vi "PID Table (Ultimate Gain and Frequency - Ziegler Nichols).vi"(5 "Control Design":u16(ring) items=["Fast", "Normal", "Slow"], 7 "Type of Controller":u16(ring)=1 items=["P", "PI", "PID"], 10 "Ultimate Period (Tu)":dbl, 11 "Ultimate Gain (Ku)":dbl) -> (1 "Derivative Time (Td)":dbl, 2 "Integral Time (Ti)":dbl, 3 "Proportional Gain (Kp)":dbl)   [LabVIEW 2017]
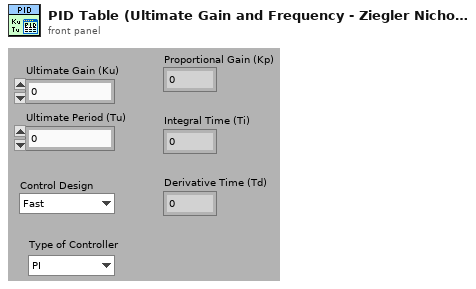
[diagram p1: front panel]
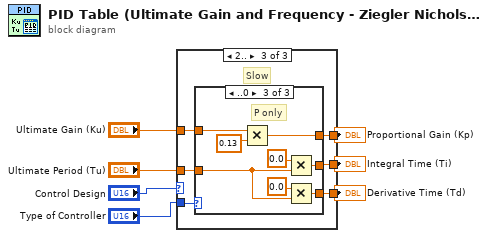
[diagram p0: block diagram]
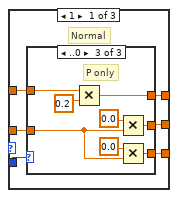
[diagram p2: hidden frame]
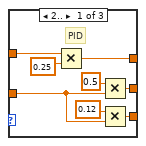
[diagram p3: hidden frame]
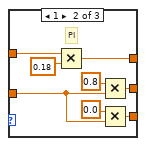
[diagram p4: hidden frame]
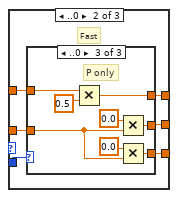
[diagram p5: hidden frame]
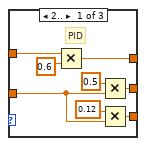
[diagram p6: hidden frame]
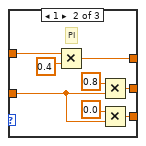
[diagram p7: hidden frame]
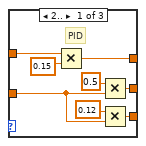
[diagram p8: hidden frame]
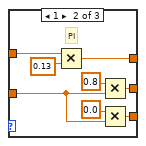
[diagram p9: hidden frame]
diagram:
  n1 = case shown="2.." "Control Design" {
    tunnel: [w13 w43 w73] -> w6
    tunnel: [w12 w42 w72] -> w7
    tunnel: [w11 w41 w71] -> w5
    tunnel: "Ultimate Period (Tu)" -> [w10 w40 w70]
    tunnel: "Ultimate Gain (Ku)" -> [w9 w39 w69]
    tunnel: "Type of Controller" -> [w8 w38 w68]
    frame 1 {
      # "Normal"
      n2 = case shown="..0" w8 {
        tunnel: [w14 w22 w30] -> w11
        tunnel: [w19 w27 w35] -> w13
        tunnel: w10 -> [w18 w26 w34]
        tunnel: [w15 w23 w31] -> w12
        tunnel: w9 -> [w16 w24 w32]
        frame 2.. {
          # "PID"
          n3 = Multiply(x=w16, y=0.25) -> (x*y=w14:dbl)
          n4 = Multiply(x=0.5, y=w18) -> (x*y=w15:dbl)
          n5 = Multiply(x=0.12, y=w18) -> (x*y=w19:dbl)
        }
        frame 1 {
          # "PI"
          n6 = Multiply(x=w24, y=0.18) -> (x*y=w22:dbl)
          n7 = Multiply(x=0.8, y=w26) -> (x*y=w23:dbl)
          n8 = Multiply(x=0.0, y=w26) -> (x*y=w27:dbl)
        }
        frame ..0 {
          # "P only"
          n9 = Multiply(x=w32, y=0.2) -> (x*y=w30:dbl)
          n10 = Multiply(x=0.0, y=w34) -> (x*y=w31:dbl)
          n11 = Multiply(x=0.0, y=w34) -> (x*y=w35:dbl)
        }
      }
    }
    frame ..0 {
      # "Fast"
      n12 = case shown="..0" w38 {
        tunnel: [w44 w52 w60] -> w41
        tunnel: [w49 w57 w65] -> w43
        tunnel: w40 -> [w48 w56 w64]
        tunnel: [w45 w53 w61] -> w42
        tunnel: w39 -> [w46 w54 w62]
        frame 2.. {
          # "PID"
          n13 = Multiply(x=w46, y=0.6) -> (x*y=w44:dbl)
          n14 = Multiply(x=0.5, y=w48) -> (x*y=w45:dbl)
          n15 = Multiply(x=0.12, y=w48) -> (x*y=w49:dbl)
        }
        frame 1 {
          # "PI"
          n16 = Multiply(x=w54, y=0.4) -> (x*y=w52:dbl)
          n17 = Multiply(x=0.8, y=w56) -> (x*y=w53:dbl)
          n18 = Multiply(x=0.0, y=w56) -> (x*y=w57:dbl)
        }
        frame ..0 {
          # "P only"
          n19 = Multiply(x=w62, y=0.5) -> (x*y=w60:dbl)
          n20 = Multiply(x=0.0, y=w64) -> (x*y=w61:dbl)
          n21 = Multiply(x=0.0, y=w64) -> (x*y=w65:dbl)
        }
      }
    }
    frame 2.. {
      # "Slow"
      n22 = case shown="..0" w68 {
        tunnel: [w74 w82 w90] -> w71
        tunnel: [w79 w87 w95] -> w73
        tunnel: w70 -> [w78 w86 w94]
        tunnel: [w75 w83 w91] -> w72
        tunnel: w69 -> [w76 w84 w92]
        frame 2.. {
          # "PID"
          n23 = Multiply(x=w76, y=0.15) -> (x*y=w74:dbl)
          n24 = Multiply(x=0.5, y=w78) -> (x*y=w75:dbl)
          n25 = Multiply(x=0.12, y=w78) -> (x*y=w79:dbl)
        }
        frame 1 {
          # "PI"
          n26 = Multiply(x=w84, y=0.13) -> (x*y=w82:dbl)
          n27 = Multiply(x=0.8, y=w86) -> (x*y=w83:dbl)
          n28 = Multiply(x=0.0, y=w86) -> (x*y=w87:dbl)
        }
        frame ..0 {
          # "P only"
          n29 = Multiply(x=w92, y=0.13) -> (x*y=w90:dbl)
          n30 = Multiply(x=0.0, y=w94) -> (x*y=w91:dbl)
          n31 = Multiply(x=0.0, y=w94) -> (x*y=w95:dbl)
        }
      }
    }
  }
  "Integral Time (Ti)" <- w7
  "Derivative Time (Td)" <- w6
  "Proportional Gain (Kp)" <- w5
